vi "Init.vi"(8 "error in (no error)":errorcluster, 11 "Agilent DSO-X 3032A in":refnum<class "Agilent DSO-X 3032A.lvclass">) -> (0 "error out":errorcluster, 3 "Agilent DSO-X 3032A out":refnum<class "Agilent DSO-X 3032A.lvclass">)   [LabVIEW 2014, in "Agilent DSO-X 3032A.lvclass"]
uses:
  Agilent DSO-X 3032A.lvclass
  Framework/Hardware/ReadoutDevice/ReadoutDevice.lvclass
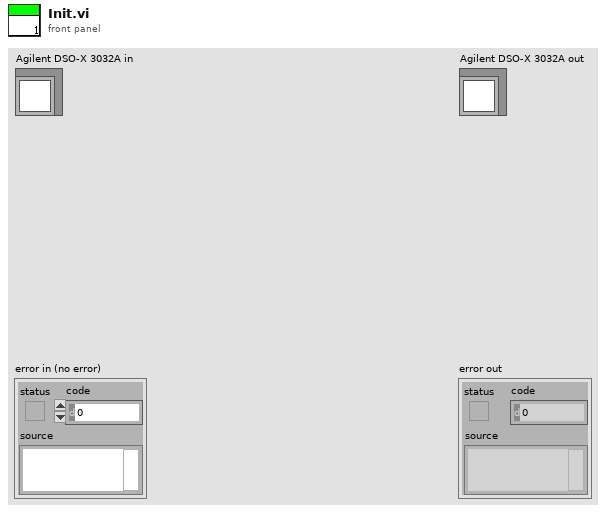
[diagram p1: front panel]
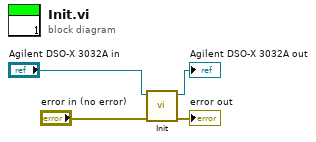
[diagram p0: block diagram]
diagram:
  n1 = call-parent "Init.vi"("error in (no error)"="error in (no error)", "Device in"="Agilent DSO-X 3032A in") -> ("error out"=→"error out":errorcluster, "Device out"=→"Agilent DSO-X 3032A out":refnum<class "Agilent DSO-X 3032A.lvclass">)  [unwired: 8 in]
